vi "Arguments - Safe Arguments if it contains key words of JKISM++.vi"() -> ()   [LabVIEW 2014]
uses:
  user.lib/_NEVSTOP/JKI State Machine++/_Support/KeyWords.vi
  user.lib/_NEVSTOP/JKI State Machine++/JKI State Machine++.lvlib
panel:
  out "Safe Argurment String":string="eaasdf->fqwvrf-&\ndddd\\\\\\\\\\not comments\n\n-@asdfvq<-1234"
  out "Origin Argurment String":string="eaasdf%2D%3Efqwvrf%2D%26%0Adddd%5C%5C%5C%5C%5Cnot comments%0A%0A%2D%40asdfvq%3C%2D1234"
  in  "Argurment String":string="eaasdf->fqwvrf-&\ndddd\\\\\\\\\\not comments\n\n, [;]\n-@asdfvq<-1234"
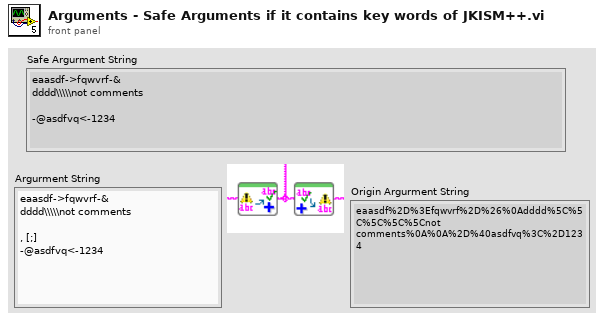
[diagram p1: front panel]
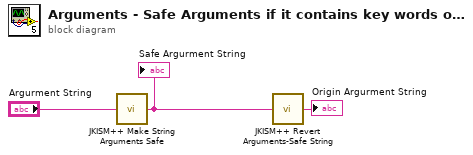
[diagram p0: block diagram]
diagram:
  n1 = call "JKISM++ Make String Arguments Safe.vi"("Argurment String"="Argurment String") -> ("Safe Argurment String"=w2:string)  [unwired: 8 in]
  "Safe Argurment String" <- w2
  n2 = call "JKISM++ Revert Arguments-Safe String.vi"("Safe Argurment String"=w2) -> ("Origin Argurment String"=→"Origin Argurment String":string)  [unwired: 8 in]
